vi "Write Test Configuration (INI) File.vi"(7 "Filename":string, 10 "FilePath in":path=path "C:/Users/Eddie.Rickey/Desktop/Test Data", 11 "Experiments":T1={"Exp 1"={"P2_Sweep_Stop_V"=36.0, "P2_Sweep_Step_V"=1.0, "Experiment Name"="", "Resistance Threshold"=1.0, "P1_Fixed_Voltage"=36.0, "P2_Sweep_Start_V"=36.0}, "Exp 3"={"P2_Sweep_Stop_V"=36.0, "P2_Sweep_Step_V"=1.0, "Experiment Name"="", "Resistance Threshold"=1.0, "P1_Fixed_Voltage"=36.0, "P2_Sweep_Start_V"=36.0}, "Exp 2"={"P2_Sweep_Stop_V"=36.0, "P2_Sweep_Step_V"=1.0, "Experiment Name"="", "Resistance Threshold"=1.0, "P1_Fixed_Voltage"=36.0, "P2_Sweep_Start_V"=36.0}, "Exp 4"={"P2_Sweep_Stop_V"=36.0, "P2_Sweep_Step_V"=1.0, "Experiment Name"="", "Resistance Threshold"=1.0, "P1_Fixed_Voltage"=36.0, "P2_Sweep_Start_V"=36.0}}) -> (3 "Final Filepath Out":path)   [LabVIEW 2013]
doc: "Setup up to 4 different experiments. During SDR setup the specific experiments will be selected."
uses:
  Support/Controls/Multiple Exp Setup.ctl
  Support/Controls/Individual User Inputs.ctl
  <vilib>/Utility/config.llb/Write Key (Double).vi
  <vilib>/Utility/config.llb/Write Key (String).vi
  <vilib>/Utility/config.llb/Write Key (Path).vi
  <vilib>/Utility/config.llb/NI_LVConfig.lvlib
panel:
  in  "Save Button":bool
  # "Test Settings"
  # "Make the Stop and Step Negative \nfor negative sweep"
  # "Calculation Settings"
  # "Test Settings"
  # "Make the Stop and Step Negative \nfor negative sweep"
  # "Calculation Settings"
  # "Test Settings"
  # "Make the Stop and Step Negative \nfor negative sweep"
  # "Calculation Settings"
  # "Test Settings"
  # "Make the Stop and Step Negative \nfor negative sweep"
  # "Calculation Settings"
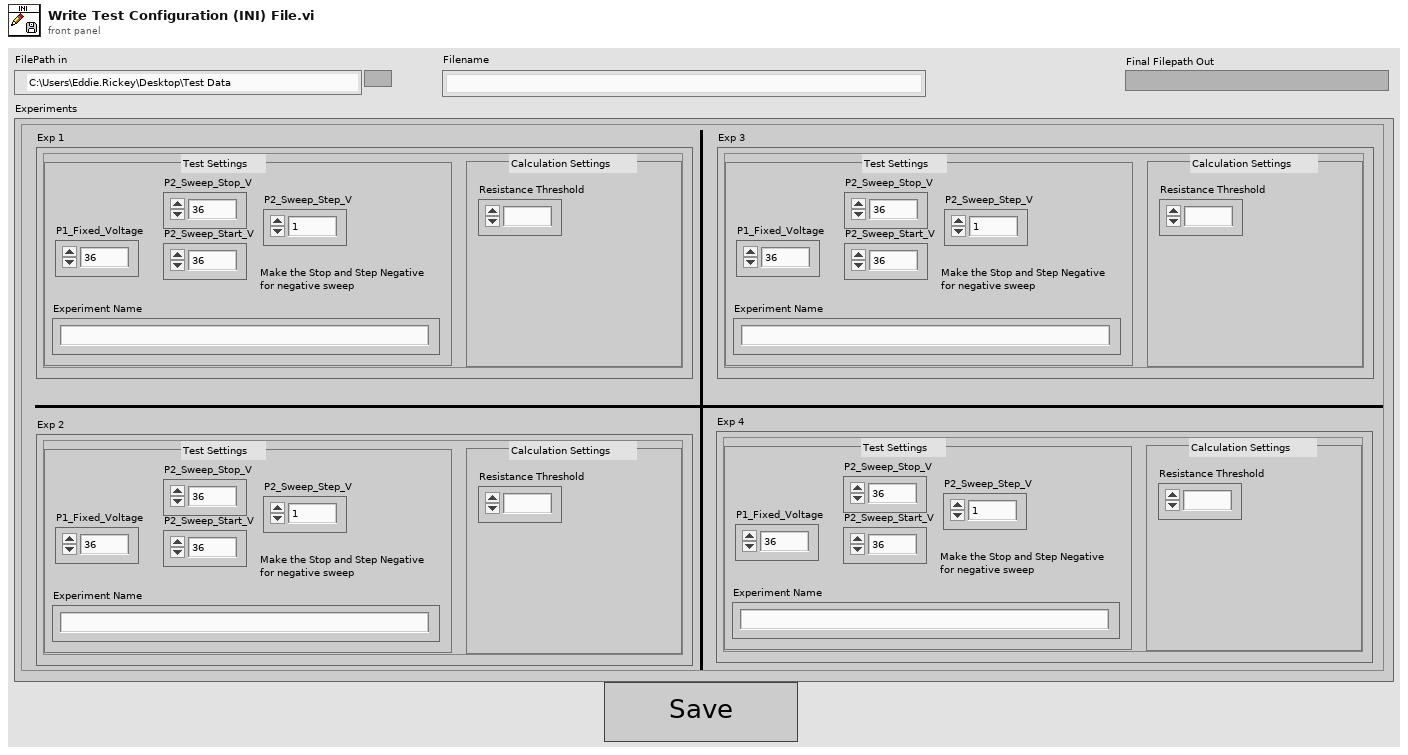
[diagram p1: front panel]
types:
  T1 = typedef "Multiple Exp Setup.ctl" = cluster{"Exp 1":T2, "Exp 3":T2, "Exp 2":T2, "Exp 4":T2}
  T2 = typedef "Individual User Inputs.ctl" = cluster{"P2_Sweep_Stop_V":dbl, "P2_Sweep_Step_V":dbl, "Experiment Name":string, "Resistance Threshold":dbl, "P1_Fixed_Voltage":dbl, "P2_Sweep_Start_V":dbl}
  T3 = typedef "NI_LVConfig.lvlib/Config Data RefNum.ctl" = refnum<k1>
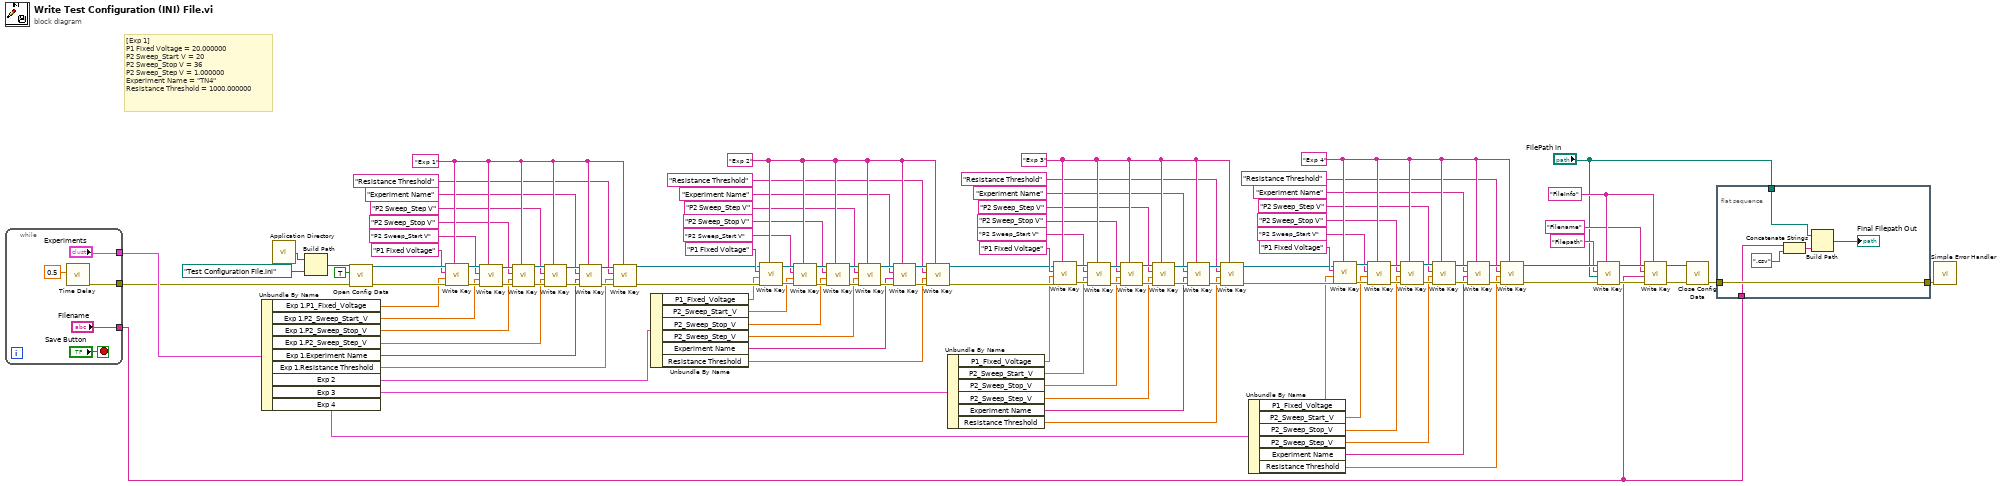
[diagram p0: block diagram]
diagram:
  w4 = "FileInfo" ("section")
  w27 = "Exp 4" ("section")
  w52 = "Exp 3" ("section")
  w79 = "Exp 2" ("section")
  w102 = "Exp 1" ("section")
  # "[Exp 1]\nP1 Fixed Voltage = 20.000000\nP2 Sweep_Start V = 20 \nP2 Sweep_Stop V = 36   \nP2 Sweep_Step V = 1.000000    \nExperiment Name = \"TN4\"\nResistance Threshold = 1000.000000"
  n1 = while {
    tunnel: ["Experiments"] -> w112
    tunnel: [w126] -> w111
    tunnel: ["Filename"] -> w1
    stop <- "Save Button" stop-if-true
    n2 = call "Time Delay"("Delay Time (s)"=0.5) -> ("error out"=w126:errorcluster)  [unwired: 10 in]
  }
  n3 = Unbundle By Name(w112) -> ("Exp 1.P1_Fixed_Voltage"=w100:dbl, "Exp 1.P2_Sweep_Start_V"=w98:dbl, "Exp 1.P2_Sweep_Stop_V"=w97:dbl, "Exp 1.P2_Sweep_Step_V"=w94:dbl, "Exp 1.Experiment Name"=w92:string, "Exp 1.Resistance Threshold"=w90:dbl, "Exp 2"=w70:T2, "Exp 3"=w63:T2, "Exp 4"=w18:T2)
  n4 = call <vilib>:"Application Directory.vi"() -> ("Application Directory"=w115:path)
  n5 = Build Path(base path=w115, name or relative path=path "Test Configuration File.ini" ("default name")) -> (appended path=w116:path)
  n6 = call <vilib>:"Open Config Data.vi"("error in (no error)"=w111, "create file if necessary (T)"=TRUE ("create file if necessary? (T)"), "configuration file path"=w116) -> ("error out"=w120:errorcluster, "refnum"=w119:T3)  [unwired: 6 in, 1 out]
  n7 = call-poly <vilib>:"Write Key.vi"("section"=w102, "error in (no error)"=w120, "value"=w100, "key"="P1 Fixed Voltage" ("Key 1"), "refnum"=w119) -> ("error out"=w108:errorcluster, "refnum out"=w107:T3)  [unwired: 4 in, 1 out]
  n8 = call-poly <vilib>:"Write Key.vi"("section"=w102, "error in (no error)"=w108, "value"=w98, "key"="P2 Sweep_Start V" ("Key 2"), "refnum"=w107) -> ("error out"=w105:errorcluster, "refnum out"=w106:T3)  [unwired: 4 in, 1 out]
  n9 = call-poly <vilib>:"Write Key.vi"("section"=w102, "error in (no error)"=w105, "value"=w97, "key"="P2 Sweep_Stop V" ("Key 2"), "refnum"=w106) -> ("error out"=w117:errorcluster, "refnum out"=w118:T3)  [unwired: 4 in, 1 out]
  n10 = call-poly <vilib>:"Write Key.vi"("section"=w102, "error in (no error)"=w117, "value"=w94, "key"="P2 Sweep_Step V" ("Key 2"), "refnum"=w118) -> ("error out"=w114:errorcluster, "refnum out"=w113:T3)  [unwired: 4 in, 1 out]
  n11 = call-poly <vilib>:"Write Key.vi"("section"=w102, "error in (no error)"=w114, "value"=w92, "key"="Experiment Name" ("Key 3"), "refnum"=w113) -> ("error out"=w104:errorcluster, "refnum out"=w103:T3)  [unwired: 4 in, 1 out]
  n12 = call-poly <vilib>:"Write Key.vi"("section"=w102, "error in (no error)"=w104, "value"=w90, "key"="Resistance Threshold" ("Key 3"), "refnum"=w103) -> ("error out"=w72:errorcluster, "refnum out"=w71:T3)  [unwired: 4 in, 1 out]
  n13 = Unbundle By Name(w70) -> ("P1_Fixed_Voltage"=w69:dbl, "P2_Sweep_Start_V"=w68:dbl, "P2_Sweep_Stop_V"=w67:dbl, "P2_Sweep_Step_V"=w66:dbl, "Experiment Name"=w65:string, "Resistance Threshold"=w64:dbl)
  n14 = call-poly <vilib>:"Write Key.vi"("section"=w79, "error in (no error)"=w72, "value"=w69, "key"="P1 Fixed Voltage" ("Key 1"), "refnum"=w71) -> ("error out"=w85:errorcluster, "refnum out"=w84:T3)  [unwired: 4 in, 1 out]
  n15 = call-poly <vilib>:"Write Key.vi"("section"=w79, "error in (no error)"=w85, "value"=w68, "key"="P2 Sweep_Start V" ("Key 2"), "refnum"=w84) -> ("error out"=w82:errorcluster, "refnum out"=w83:T3)  [unwired: 4 in, 1 out]
  n16 = call-poly <vilib>:"Write Key.vi"("section"=w79, "error in (no error)"=w82, "value"=w67, "key"="P2 Sweep_Stop V" ("Key 2"), "refnum"=w83) -> ("error out"=w88:errorcluster, "refnum out"=w89:T3)  [unwired: 4 in, 1 out]
  n17 = call-poly <vilib>:"Write Key.vi"("section"=w79, "error in (no error)"=w88, "value"=w66, "key"="P2 Sweep_Step V" ("Key 2"), "refnum"=w89) -> ("error out"=w87:errorcluster, "refnum out"=w86:T3)  [unwired: 4 in, 1 out]
  n18 = call-poly <vilib>:"Write Key.vi"("section"=w79, "error in (no error)"=w87, "value"=w65, "key"="Experiment Name" ("Key 3"), "refnum"=w86) -> ("error out"=w81:errorcluster, "refnum out"=w80:T3)  [unwired: 4 in, 1 out]
  n19 = call-poly <vilib>:"Write Key.vi"("section"=w79, "error in (no error)"=w81, "value"=w64, "key"="Resistance Threshold" ("Key 3"), "refnum"=w80) -> ("error out"=w45:errorcluster, "refnum out"=w44:T3)  [unwired: 4 in, 1 out]
  n20 = Unbundle By Name(w63) -> ("P1_Fixed_Voltage"=w43:dbl, "P2_Sweep_Start_V"=w42:dbl, "P2_Sweep_Stop_V"=w41:dbl, "P2_Sweep_Step_V"=w40:dbl, "Experiment Name"=w39:string, "Resistance Threshold"=w38:dbl)
  n21 = call-poly <vilib>:"Write Key.vi"("section"=w52, "error in (no error)"=w45, "value"=w43, "key"="P1 Fixed Voltage" ("Key 1"), "refnum"=w44) -> ("error out"=w58:errorcluster, "refnum out"=w57:T3)  [unwired: 4 in, 1 out]
  n22 = call-poly <vilib>:"Write Key.vi"("section"=w52, "error in (no error)"=w58, "value"=w42, "key"="P2 Sweep_Start V" ("Key 2"), "refnum"=w57) -> ("error out"=w55:errorcluster, "refnum out"=w56:T3)  [unwired: 4 in, 1 out]
  n23 = call-poly <vilib>:"Write Key.vi"("section"=w52, "error in (no error)"=w55, "value"=w41, "key"="P2 Sweep_Stop V" ("Key 2"), "refnum"=w56) -> ("error out"=w61:errorcluster, "refnum out"=w62:T3)  [unwired: 4 in, 1 out]
  n24 = call-poly <vilib>:"Write Key.vi"("section"=w52, "error in (no error)"=w61, "value"=w40, "key"="P2 Sweep_Step V" ("Key 2"), "refnum"=w62) -> ("error out"=w60:errorcluster, "refnum out"=w59:T3)  [unwired: 4 in, 1 out]
  n25 = call-poly <vilib>:"Write Key.vi"("section"=w52, "error in (no error)"=w60, "value"=w39, "key"="Experiment Name" ("Key 3"), "refnum"=w59) -> ("error out"=w54:errorcluster, "refnum out"=w53:T3)  [unwired: 4 in, 1 out]
  n26 = call-poly <vilib>:"Write Key.vi"("section"=w52, "error in (no error)"=w54, "value"=w38, "key"="Resistance Threshold" ("Key 3"), "refnum"=w53) -> ("error out"=w20:errorcluster, "refnum out"=w19:T3)  [unwired: 4 in, 1 out]
  n27 = Unbundle By Name(w18) -> ("P1_Fixed_Voltage"=w17:dbl, "P2_Sweep_Start_V"=w16:dbl, "P2_Sweep_Stop_V"=w15:dbl, "P2_Sweep_Step_V"=w14:dbl, "Experiment Name"=w13:string, "Resistance Threshold"=w12:dbl)
  n28 = call-poly <vilib>:"Write Key.vi"("section"=w27, "error in (no error)"=w20, "value"=w17, "key"="P1 Fixed Voltage" ("Key 1"), "refnum"=w19) -> ("error out"=w33:errorcluster, "refnum out"=w32:T3)  [unwired: 4 in, 1 out]
  n29 = call-poly <vilib>:"Write Key.vi"("section"=w27, "error in (no error)"=w33, "value"=w16, "key"="P2 Sweep_Start V" ("Key 2"), "refnum"=w32) -> ("error out"=w30:errorcluster, "refnum out"=w31:T3)  [unwired: 4 in, 1 out]
  n30 = call-poly <vilib>:"Write Key.vi"("section"=w27, "error in (no error)"=w30, "value"=w15, "key"="P2 Sweep_Stop V" ("Key 2"), "refnum"=w31) -> ("error out"=w36:errorcluster, "refnum out"=w37:T3)  [unwired: 4 in, 1 out]
  n31 = call-poly <vilib>:"Write Key.vi"("section"=w27, "error in (no error)"=w36, "value"=w14, "key"="P2 Sweep_Step V" ("Key 2"), "refnum"=w37) -> ("error out"=w35:errorcluster, "refnum out"=w34:T3)  [unwired: 4 in, 1 out]
  n32 = call-poly <vilib>:"Write Key.vi"("section"=w27, "error in (no error)"=w35, "value"=w13, "key"="Experiment Name" ("Key 3"), "refnum"=w34) -> ("error out"=w29:errorcluster, "refnum out"=w28:T3)  [unwired: 4 in, 1 out]
  n33 = call-poly <vilib>:"Write Key.vi"("section"=w27, "error in (no error)"=w29, "value"=w12, "key"="Resistance Threshold" ("Key 3"), "refnum"=w28) -> ("error out"=w11:errorcluster, "refnum out"=w6:T3)  [unwired: 4 in, 1 out]
  n34 = call-poly <vilib>:"Write Key.vi"("section"=w4, "error in (no error)"=w11, "value"="FilePath in", "key"="Filepath" ("Key 1"), "refnum"=w6) -> ("error out"=w10:errorcluster, "refnum out"=w7:T3)  [unwired: 4 in, 1 out]
  n35 = call-poly <vilib>:"Write Key.vi"("section"=w4, "error in (no error)"=w10, "value"=w1, "key"="Filename" ("Key 1"), "refnum"=w7) -> ("error out"=w9:errorcluster, "refnum out"=w8:T3)  [unwired: 4 in, 1 out]
  n36 = call <vilib>:"Close Config Data.vi"("error in (no error)"=w9, "refnum"=w8) -> ("error out"=w110:errorcluster)  [unwired: 1 in, 8 out]
  n37 = flat-sequence {
    tunnel: w110 -> [w132]
    tunnel: [w132] -> w109
    tunnel: "FilePath in" -> [w131]
    tunnel: w1 -> [w128]
    frame #0 {
      n38 = Concatenate Strings(w128, ".csv" ("string")) -> (w130:string)
      n39 = Build Path(base path=w131, name or relative path=w130) -> (appended path=→"Final Filepath Out":path)
    }
  }
  n40 = call <vilib>:"Simple Error Handler.vi"("error in (no error)"=w109) -> ()  [unwired: 2 in, 7 out]
